vi "2D Array Decimate.vi"(8 "averaging":bool=TRUE, 9 "y decimating factor":dbl=1.0, 10 "x decimating factor":dbl=1.0, 11 "Input 2D Array":dbl[][](array[numeric])) -> (1 "y dim":u32, 2 "x dim":u32, 3 "output array":dbl[][](array[numeric]))   [LabVIEW 2018]
uses:
  <vilib>/Analysis/2dsp.llb/Decimate (single shot, DBL).vi
  <vilib>/Analysis/NI_AALPro.lvlib
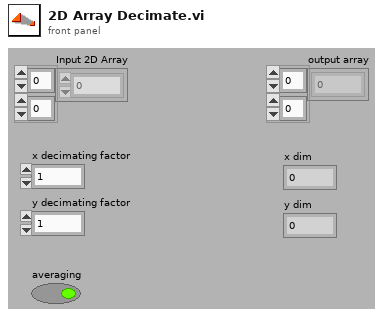
[diagram p1: front panel]
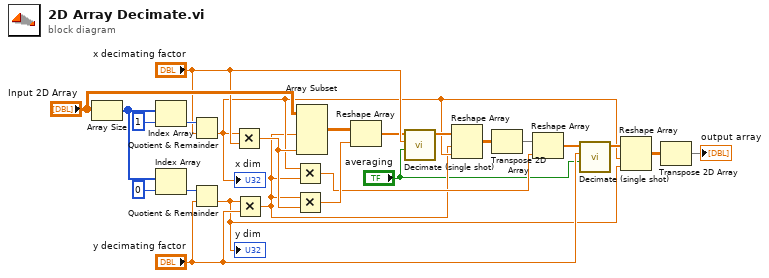
[diagram p0: block diagram]
diagram:
  n1 = Array Size(array="Input 2D Array") -> (size(s)=w22:i32[])
  n2 = Index Array(array=w22, index=1) -> (element=w21:i32)
  n3 = Index Array(array=w22, index=0) -> (element=w17:i32)
  n4 = Quotient & Remainder(x=w21, y="x decimating factor") -> (floor(x/y)=w3:dbl)  [unwired: 1 out]
  "x dim" <- w3
  n5 = Quotient & Remainder(x=w17, y="y decimating factor") -> (floor(x/y)=w7:dbl)  [unwired: 1 out]
  "y dim" <- w7
  n6 = Multiply(x=w3, y="x decimating factor") -> (x*y=w9:dbl)
  n7 = Multiply(x=w7, y="y decimating factor") -> (x*y=w2:dbl)
  n8 = Multiply(x=w3, y=w2) -> (x*y=w4:dbl)
  n9 = Multiply(x=w2, y=w9) -> (x*y=w10:dbl)
  n10 = Array Subset(array="Input 2D Array", length (row)=w2, length (col)=w9) -> (w19:dbl[][])  [unwired: 2 in]
  n11 = Reshape Array(w19, w10) -> (w11:dbl[])
  n12 = call-poly <vilib>:"Decimate (single shot).vi"("averaging"="averaging", "decimating factor"="x decimating factor", "X"=w11) -> ("Decimated Array"=w18:dbl[])  [unwired: 8 out]
  n13 = Reshape Array(w18, w2, w3) -> (w16:dbl[][])
  n14 = Transpose 2D Array(2D array=w16) -> (transposed array=w8:dbl[][])
  n15 = Reshape Array(w8, w4) -> (w15:dbl[])
  n16 = call-poly <vilib>:"Decimate (single shot).vi"("averaging"="averaging", "decimating factor"="y decimating factor", "X"=w15) -> ("Decimated Array"=w14:dbl[])  [unwired: 8 out]
  n17 = Reshape Array(w14, w3, w7) -> (w6:dbl[][])
  n18 = Transpose 2D Array(2D array=w6) -> (transposed array=→"output array":dbl[][])
